vi "Utility - Check Hardware etc.vi"(7 "error in":errorcluster) -> (0 "error out":errorcluster, 2 "OK?":bool)   [LabVIEW 2014]
doc: "Queue Reference:\n\nDefines name queue references for each of the queued state machines. This includes a custom control for both the queue data type (cluster) and a custer of all the queue refnums."
uses:
  FileIO/TypeDef - File Actions.ctl
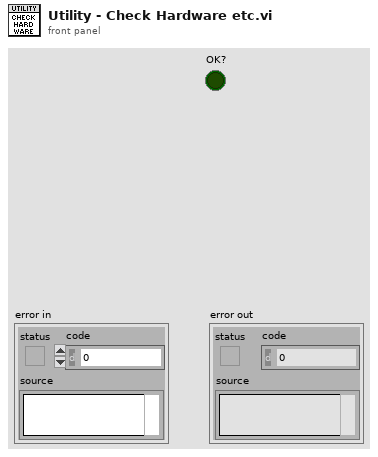
[diagram p1: front panel]
types:
  T1 = typedef "TypeDef - File Actions.ctl" = enum16{"Read", "Write", "Get Current"}
  T2 = typedef "TypeDef - System Configuration.ctl" = cluster{"Results FilePath":path, "Analysis Parameters":cluster{"Area":cluster{"Lower Value":dbl, "Upper Value":dbl}, "Circle Filter Radius":cluster{"Lower Value":sgl, "Upper Value":sgl}, "Edge Detection Threshold":u16}, "ROI Parameters":cluster{"ROI size (in Radius)":cluster{"Width":dbl, "Height":dbl}}}
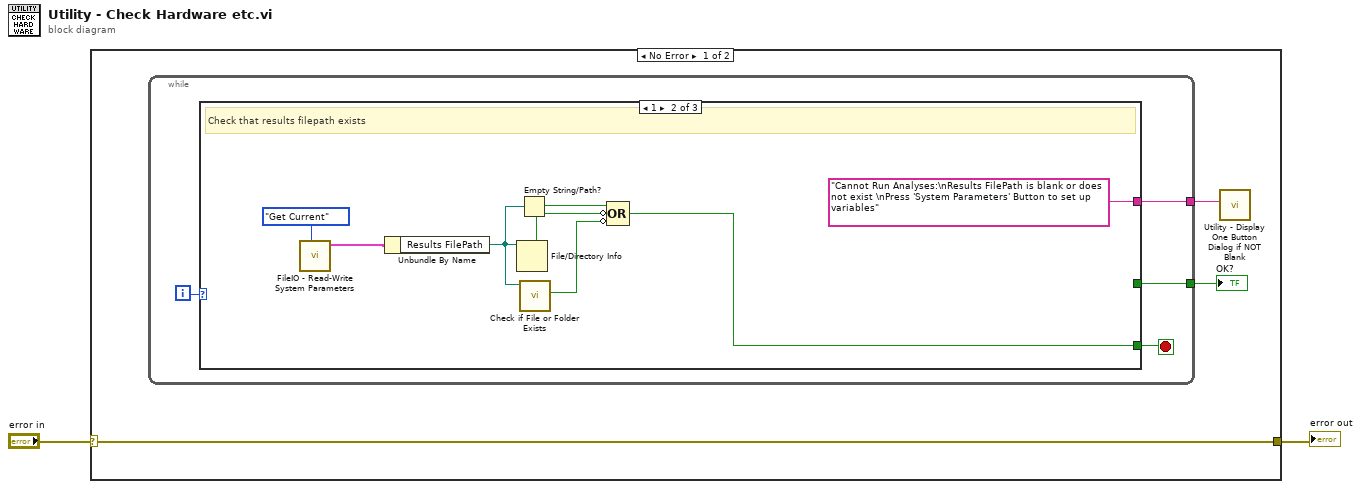
[diagram p0: block diagram]
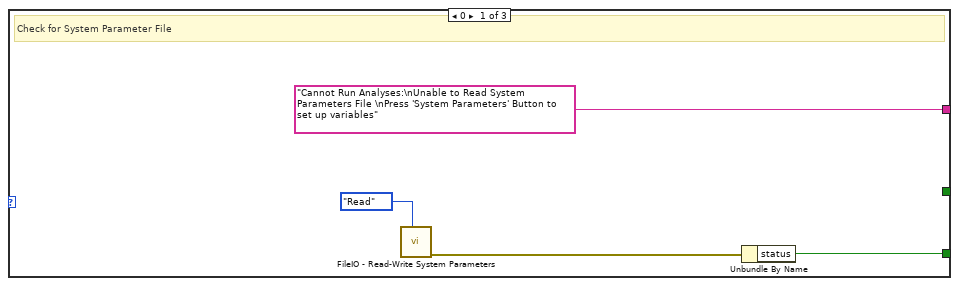
[diagram p2: hidden frame]
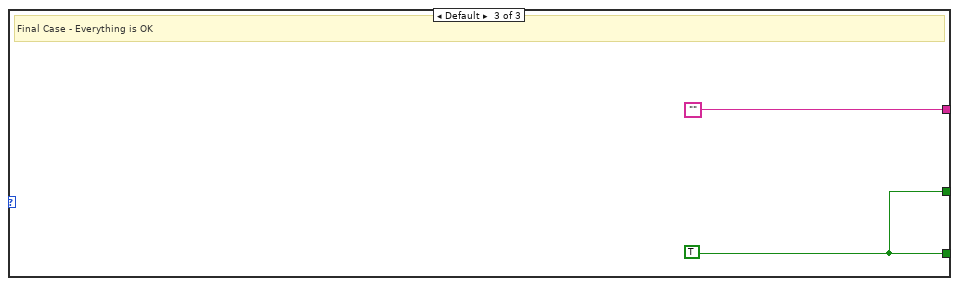
[diagram p3: hidden frame]
diagram:
  n1 = case shown="No Error" "error in" {
    selector: "error in" -> [w3 w24]
    tunnel: [w3 w24] -> w1
    frame No Error {
      n2 = while {
        tunnel: [w7] -> w5
        tunnel: [w6] -> w4
        i -> [w9]
        stop <- w8 stop-if-true
        n3 = case shown="1" w9 {
          tunnel: [w13 w14 w22] -> w8
          tunnel: ["Cannot Run Analyses:\nUnable to Read System Parameters File \nPress 'System Parameters' Button to set up variables" "Cannot Run Analyses:\nResults FilePath is blank or does not exist \nPress 'System Parameters' Button to set up variables" ""] -> w7
          tunnel: [_ _ w22] -> w6
          frame 0 {
            # "Check for System Parameter File"
            n4 = call "FileIO - Read-Write System Parameters.vi"("Action"=TypeDef_-_File_Actions."Read") -> ("error out"=w12:errorcluster)  [unwired: 9 in, 1 out]
            n5 = Unbundle By Name(w12) -> ("status"=w13:bool)
          }
          frame 1 {
            # "Check that results filepath exists"
            n6 = call "FileIO - Read-Write System Parameters.vi"("Action"=TypeDef_-_File_Actions."Get Current") -> ("System Parameters out"=w15:T2)  [unwired: 9 in, 1 out]
            n7 = Unbundle By Name(w15) -> ("Results FilePath"=w17:path)
            n8 = File/Directory Info(path=w17) -> (directory=w18:bool)  [unwired: 1 in, 6 out]
            n9 = Empty String/Path?(string/path=w17) -> (empty?=w19:bool)
            n10 = call <vilib>:"Check if File or Folder Exists.vi"("path"=w17) -> ("file or folder exists?"=w16:bool)  [unwired: 8 in, 2 out]
            n11 = Compound Arithmetic op=OR(w19, invert w18, invert w16) -> (w14:bool)
          }
          frame Default {
            w22 = TRUE
            # "Final Case - Everything is OK"
          }
        }
      }
      "OK?" <- w4
      n12 = call "Utility - Display One Button Dialog if NOT Blank.vi"("message"=w5) -> ()  [unwired: 10 in, 1 out]
    }
    frame Error {
    }
  }
  "error out" <- w1
